vi "Build Message with Arguments(Auto Check).vi"(5 "State With Arguments":string, 7 "Arguments (\"\")":string, 9 "Target Module (\"\")":string) -> (6 "CSM Message String":string)   [LabVIEW 2017, in "Communicable State Machine.lvlib"]
doc: "Concatenates and generates CSM message strings. The message type symbol is automatically detected based on the input <b>State with Arguments</b>.\n\n\n> [!NOTE] <b>Message Building API</b>\n>\n> This type of API is only used to concatenate message strings and does not send messages directly. The strings need to be merged into the CSM state queue, and the messages will be sent and the operation executed within the Parse State Queue++ VI. If you are familiar with CSM rules, you do not need to use this type of API. You can type the corresponding message string or operation string directly into the string.\n\n\n> [!NOTE] <b>CSM Message Target Module Description</b>\n>\n> In Normal Mode, the target module for a CSM message is the specified module name.\n> System-level modules start with a `.` in their name. The target module for a CSM message includes the `.` in the name. For example, if the requested module name is `.System`, the target module for the CSM message is `.System`.\n> In Worker Mode, the target module for a CSM message can only be the overall module name, not the node name. For example, if the requested module name is `Worker#`, the target module for the CSM message is `Worker`.\n> In Chain of Responsibility Mode, the target module for a CSM message can only be the overall module name, not the node name. For example, if the requested module name is `Chain$1`, the target module for the CSM message is `Chain`.\n> In Chain of Responsibility Mode, a message is routed directly based on handling capability and priority (smaller number = higher priority) and is not passed sequentially across nodes.\n\n\n-- <b>Controls</b> --\n- <b>State with Arguments</b>: CSM state string, which can contain arguments and target module information.\n- <b>Arguments (\"\")</b>: Argument information. Arguments contained in <b>State with Arguments</b> will be replaced.\n- <b>Target Module (\"\")</b>: Target module. If empty, the default module in <b>State with Arguments</b> will be used.\n\n-- <b>Indicators</b> --\n- <b>CSM Message String</b>: Concatenated CSM message string."
uses:
  Communicable State Machine.lvlib
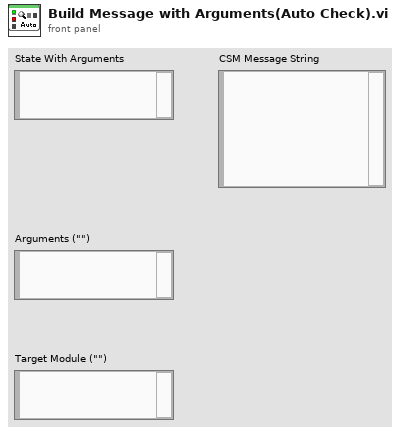
[diagram p1: front panel]
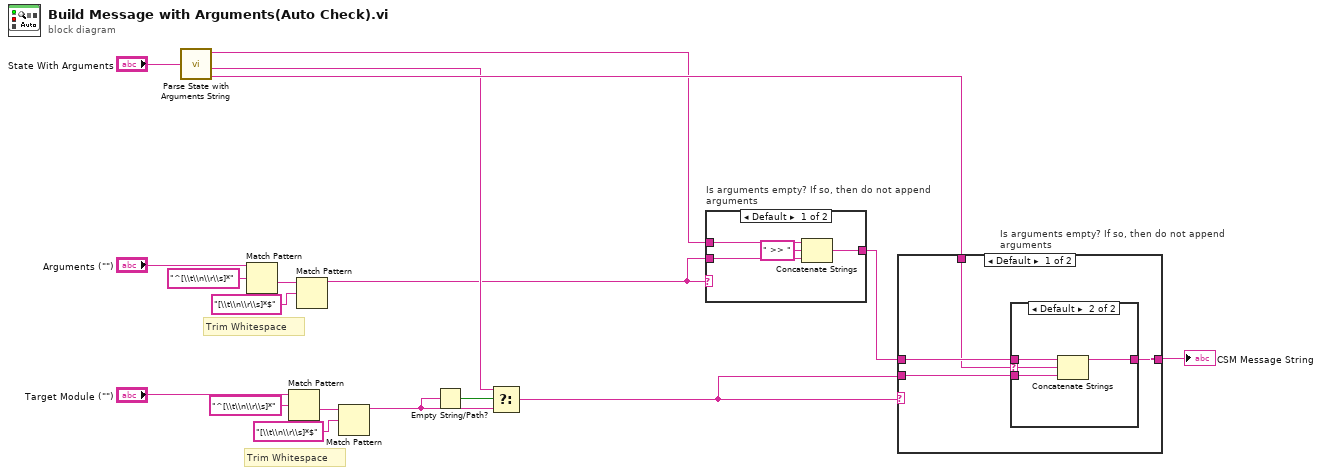
[diagram p0: block diagram]
diagram:
  # "Trim Whitespace"
  # "Trim Whitespace"
  n1 = call "Parse State with Arguments String.vi"("State With Arguments"="State With Arguments") -> ("State"=w2:string, "Target Module"=w6:string, "Message Symbol"=w8:string)  [unwired: 6 in, 1 out]
  n2 = Match Pattern(string="Arguments (\"\")", regular expression="^[\\t\\n\\r\\s]*") -> (after substring=w17:string)  [unwired: 1 in, 3 out]
  n3 = Match Pattern(string="Target Module (\"\")", regular expression="^[\\t\\n\\r\\s]*") -> (after substring=w13:string)  [unwired: 1 in, 3 out]
  n4 = Match Pattern(string=w17, regular expression="[\\t\\n\\r\\s]*$") -> (before substring=w1:string)  [unwired: 1 in, 3 out]
  n5 = Match Pattern(string=w13, regular expression="[\\t\\n\\r\\s]*$") -> (before substring=w4:string)  [unwired: 1 in, 3 out]
  n6 = Empty String/Path?(string/path=w4) -> (empty?=w7:bool)
  n7 = Select(t=w6, s=w7, f=w4) -> (s? t:f=w3:string)
  n8 = case "Is arguments empty? If so, then do not append arguments" shown="Default" w1 {
    tunnel: [w19 w23] -> w10
    tunnel: w2 -> [w22 w23]
    tunnel: w1 -> [w20 _]
    frame Default {
      n9 = Concatenate Strings(w22, " >> " ("string"), w20) -> (w19:string)
    }
    frame "" {
    }
  }
  n10 = case "Is arguments empty? If so, then do not append arguments" shown="Default" w3 {
    tunnel: [w25 w33] -> w11
    tunnel: w10 -> [w27 w33]
    tunnel: w3 -> [w26 _]
    tunnel: w8 -> [w24 _]
    frame Default {
      n11 = case shown="Default" w24 {
        selector: w24 -> [_ w29]
        tunnel: w27 -> [w28 w32]
        tunnel: w26 -> [_ w31]
        tunnel: [w28 w30] -> w25
        frame "" {
        }
        frame Default {
          n12 = Concatenate Strings(w32, w29, w31) -> (w30:string)
        }
      }
    }
    frame "" {
    }
  }
  "CSM Message String" <- w11
